vi "Generate Tag Clusters.vi"(9 "NI Skyline Tag in":refnum<class "NI Skyline Tag.lvclass">, 10 "HTTP Output in":T1[](array[typedef]), 11 "AMQP output in":T1[](array[typedef])) -> (0 "Index":i32, 1 "AMQP":bool, 2 "HTTP Output out":T1[](array[typedef]), 3 "AMQP output out":T1[](array[typedef]))   [LabVIEW 2015, in "SystemLink runtime.lvclass"]
uses:
  SystemLink runtime.lvclass
  <vilib>/Skyline/Tag/Wrapper/Wrapper_class/Tag Value Cluster Wrapper.ctl
  <vilib>/Skyline/Configuration/Configuration_class/NI Skyline Configuration.lvclass
  <vilib>/Skyline/Tag/Shared/typedefs/Tag Value Cluster.ctl
  <vilib>/Skyline/Tag/Shared/typedefs/DataType.ctl
  <vilib>/Skyline/Tag/Wrapper/Wrapper_class/NI Skyline Tag.lvclass
  <vilib>/Skyline/Configuration/Configuration AMQP_class/NI Skyline Configuration AMQP.lvclass
  <vilib>/Skyline/Configuration/Configuration HTTP_class/NI Skyline Configuration HTTP.lvclass
  <vilib>/Skyline/Tag/Wrapper/Wrapper_class/Generate Tag Cluster (DBL) 2.vi
  <vilib>/Skyline/Tag/Wrapper/Wrapper_class/Generate Tag Cluster (String) 2.vi
  <vilib>/Skyline/Tag/Wrapper/Wrapper_class/Generate Tag Cluster (Boolean) 2.vi
  <vilib>/Skyline/Tag/Wrapper/Wrapper_class/Generate Tag Cluster (I32) 2.vi
  <vilib>/Skyline/Tag/Shared/NI Skyline Tag.lvlib
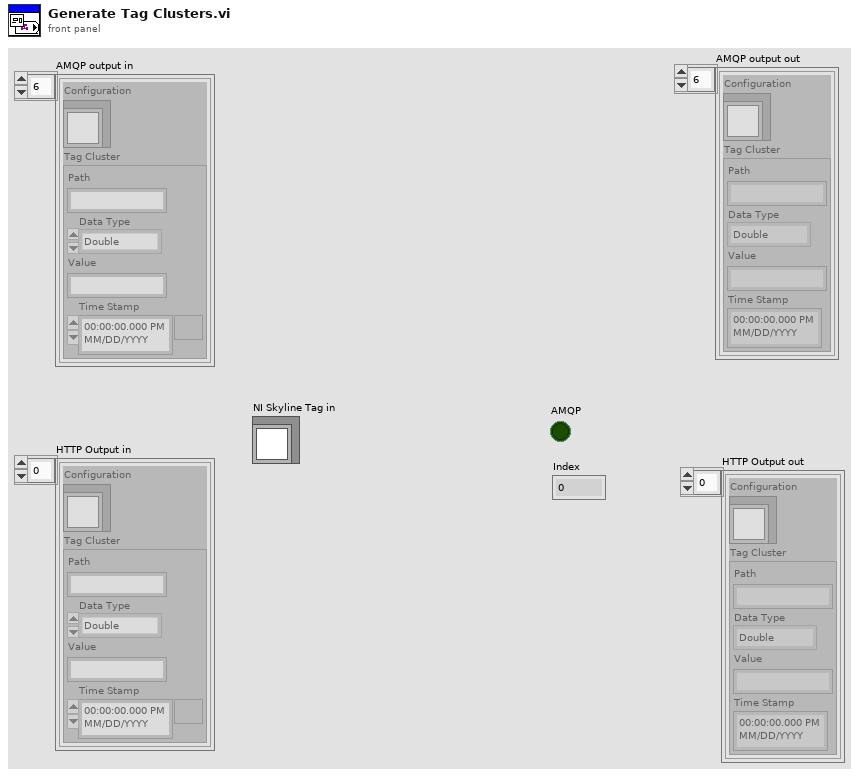
[diagram p1: front panel]
types:
  T1 = typedef "NI Skyline Tag.lvclass/Tag Value Cluster Wrapper.ctl" = cluster{"Configuration":refnum<class "NI Skyline Configuration.lvclass">, "Tag Cluster":T2}
  T2 = typedef "NI Skyline Tag.lvlib/Tag Value Cluster.ctl" = cluster{"Path":string, "Data Type":T3, "Value":string, "Time Stamp":timestamp}
  T3 = typedef "NI Skyline Tag.lvlib/DataType.ctl" = enum32{"Double", "I32", "String", "Boolean", "U64", "Timestamp"}
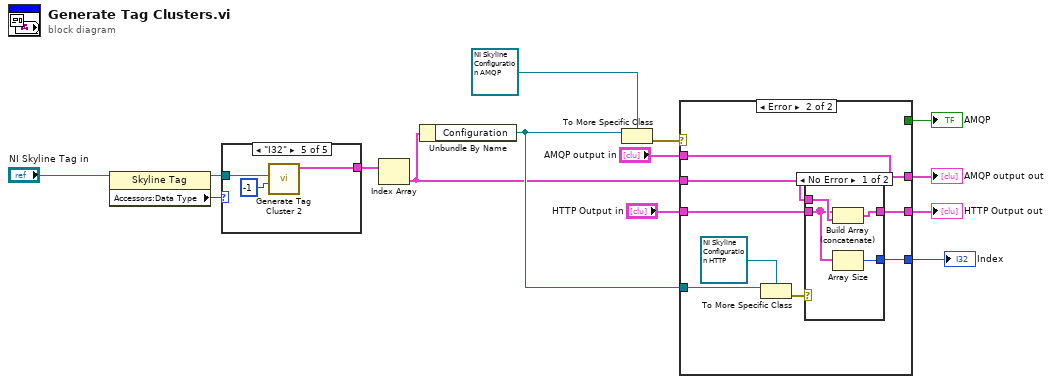
[diagram p0: block diagram]
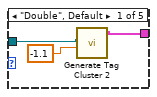
[diagram p2: hidden frame]
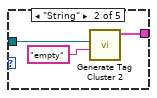
[diagram p3: hidden frame]
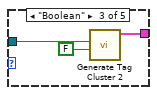
[diagram p4: hidden frame]
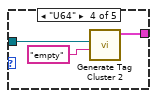
[diagram p5: hidden frame]
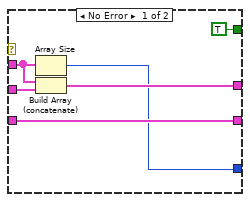
[diagram p6: hidden frame]
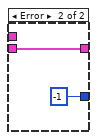
[diagram p7: hidden frame]
diagram:
  n1 = property class="Skyline Tag"(reference="NI Skyline Tag in") -> (reference out=w1:refnum<class "NI Skyline Tag.lvclass">, "Accessors:Data Type"=w2:T3)  [unwired: 1 in, 1 out]
  n2 = case shown="\"I32\"" w2 {
    tunnel: w1 -> [w16 w18 w22 w24 w29]
    tunnel: [w17 w20 w23 w26 w28] -> w8
    frame "Double", Default {
      n3 = call-poly <vilib>:"Generate Tag Cluster 2.vi"("value"=-1.1, "tag in"=w16) -> ("tag clusters out"=w17:T1[])  [unwired: 7 in, 2 out]
    }
    frame "String" {
      n4 = call-poly <vilib>:"Generate Tag Cluster 2.vi"("value"="empty", "tag in"=w18) -> ("tag clusters out"=w20:T1[])  [unwired: 7 in, 2 out]
    }
    frame "Boolean" {
      n5 = call-poly <vilib>:"Generate Tag Cluster 2.vi"("value"=FALSE, "tag in"=w22) -> ("tag clusters out"=w23:T1[])  [unwired: 7 in, 2 out]
    }
    frame "U64" {
      n6 = call-poly <vilib>:"Generate Tag Cluster 2.vi"("value"="empty", "tag in"=w24) -> ("tag clusters out"=w26:T1[])  [unwired: 7 in, 2 out]
    }
    frame "I32" {
      n7 = call-poly <vilib>:"Generate Tag Cluster 2.vi"("value"=-1, "tag in"=w29) -> ("tag clusters out"=w28:T1[])  [unwired: 7 in, 2 out]
    }
  }
  n8 = Index Array(array=w8) -> (element=w6:T1)  [unwired: 1 in]
  n9 = Unbundle By Name(w6) -> ("Configuration"=w7:refnum<class "NI Skyline Configuration.lvclass">)
  n10 = To More Specific Class(target class=refnum<class "NI Skyline Configuration AMQP.lvclass"> refnum ("AMQP Configuration"), reference=w7) -> (error out=w9:errorcluster)  [unwired: 1 in, 1 out]
  n11 = case shown="Error" w9 {
    tunnel: w6 -> [w35 w39]
    tunnel: "AMQP output in" -> [w31 w43]
    tunnel: "HTTP Output in" -> [w33 w41]
    tunnel: [w34 w43] -> w12
    tunnel: [w33 w40] -> w14
    tunnel: w7 -> [_ w37]
    tunnel: [TRUE ("AMQP") _] -> w5
    tunnel: [w30 w36] -> w4
    frame No Error {
      n12 = Array Size(array=w31) -> (size(s)=w30:i32)
      n13 = Build Array (concatenate)(w31, w35) -> (w34:T1[])
    }
    frame Error {
      n14 = To More Specific Class(target class=refnum<class "NI Skyline Configuration HTTP.lvclass"> refnum ("HTTP Configuration"), reference=w37) -> (error out=w42:errorcluster)  [unwired: 1 in, 1 out]
      n15 = case shown="No Error" w42 {
        tunnel: w41 -> [w45 w49]
        tunnel: [w47 w49] -> w40
        tunnel: w39 -> [w46 _]
        tunnel: [w44 -1] -> w36
        frame No Error {
          n16 = Build Array (concatenate)(w45, w46) -> (w47:T1[])
          n17 = Array Size(array=w45) -> (size(s)=w44:i32)
        }
        frame Error {
        }
      }
    }
  }
  "HTTP Output out" <- w14
  "AMQP output out" <- w12
  "AMQP" <- w5
  "Index" <- w4
